vi "Get Frame Position (Index).vi"(8 "error in (no error)":errorcluster, 11 "Reader in":refnum<class "Reader.lvclass">) -> (0 "error out":errorcluster, 2 "Index":u64, 3 "Reader":refnum<class "Reader.lvclass">)   [LabVIEW 2020, in "video_io.lvlib" / "Reader.lvclass"]
uses:
  Reader.lvclass
  Reader.lvclass/Reader.ctl
  acb2feee-aaa4-4f40-955f-c8ac8e9dff35.vi
  <vilib>/Utility/error.llb/Error Cluster From Error Code.vi
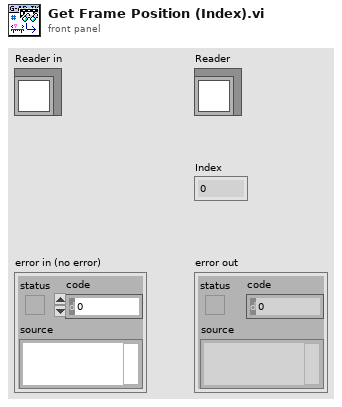
[diagram p1: front panel]
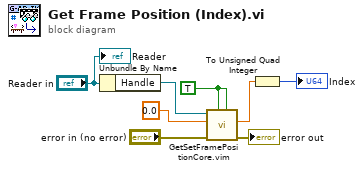
[diagram p0: block diagram]
diagram:
  w3 = TRUE ("Get")
  n1 = Unbundle By Name("Reader in") -> ("Handle"=w8:refnum<data-value>)
  n2 = call "GetSetFramePositionCore.vim"("As Frame Index"=w3, "Get"=w3, "error in (no error)"="error in (no error)", "Position In"=0.0, "Handle"=w8) -> ("error out"=→"error out":errorcluster, "Position Out"=w2:dbl)  [unwired: 5 in]
  n3 = To Unsigned Quad Integer(1:w2) -> (0:→"Index":u64)
  "Reader" <- "Reader in"
